vi "oa_TV Decimate N (NChan).vi"(5 "reset? (F)":bool, 8 "error in (no error)":errorcluster, 10 "pulse/revolution":i32[](array[numeric]), 11 "pulse position [s]":cluster{dbl[]}[](array[cluster]) {"?" format="%.2f"}) -> (0 "error out":errorcluster, 1 "revulotion index":i32[](array[numeric]), 2 "revulotion":i32[](array[numeric]), 3 "pulse positions":cluster{dbl[]}[](array[cluster]))   [LabVIEW 2017, in "SoundVib_Torsional.lvlib"]
uses:
  <vilib>/addons/Sound and Vibration/Order Analysis/Torsional Vibration/SoundVib_Torsional.lvlib
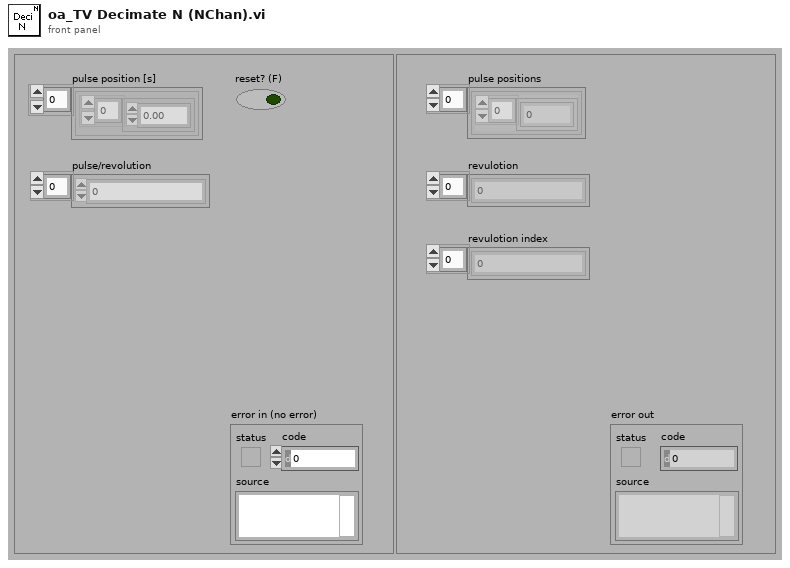
[diagram p1: front panel]
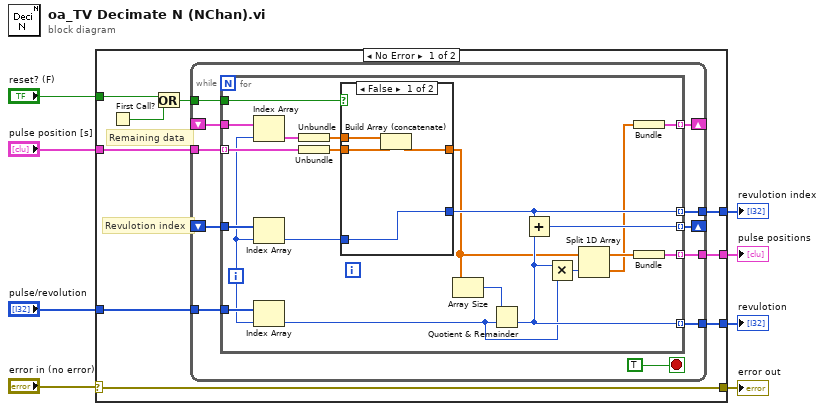
[diagram p0: block diagram]
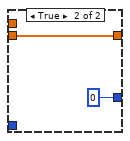
[diagram p2: hidden frame]
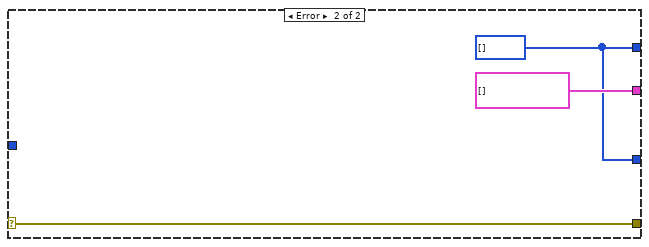
[diagram p3: hidden frame]
diagram:
  n1 = case shown="No Error" "error in (no error)" {
    selector: "error in (no error)" -> [w17 w58]
    tunnel: [w17 w58] -> w7
    tunnel: "pulse/revolution" -> [w16 _]
    tunnel: [w12 cluster{dbl[]}[] []] -> w5
    tunnel: [w15 w56] -> w4
    tunnel: "pulse position [s]" -> [w11 _]
    tunnel: [w10 w56] -> w2
    tunnel: "reset? (F)" -> [w9 _]
    frame No Error {
      # "Revulotion index"
      # "Remaining data"
      n2 = First Call?() -> (First Call?: T/F=w14:bool)
      n3 = Or(x=w9, y=w14) -> (x .or. y?=w13:bool)
      n4 = while {
        tunnel: w16 -> [w23]
        tunnel: [w24] -> w15
        tunnel: w13 -> [w28]
        shift-right: [w18] -> _
        shift-left: _ -> [w27]
        shift-right: [w26] -> _
        shift-left: _ -> [w25]
        tunnel: [w22] -> w12
        tunnel: [w21] -> w10
        tunnel: w11 -> [w19]
        stop <- TRUE stop-if-true
        n5 = for {
          tunnel: w28 -> [w48]
          tunnel: w19 -> [w43] mode=indexing
          tunnel: w27 -> [w38]
          tunnel: [w47] -> w26 mode=indexing
          tunnel: w25 -> [w37]
          tunnel: [w46] -> w24 mode=indexing
          tunnel: [w31] -> w18 mode=indexing
          tunnel: w23 -> [w36]
          tunnel: [w39] -> w22 mode=indexing
          tunnel: [w44] -> w21 mode=indexing
          i -> [w34]
          n6 = Index Array(array=w38, index=w34) -> (element=w30:cluster{dbl[]})
          n7 = Index Array(array=w37, index=w34) -> (element=w33:i32)
          n8 = Index Array(array=w36, index=w34) -> (element=w35:i32)
          n9 = Unbundle(w30) -> (w29:dbl[])
          n10 = Unbundle(w43) -> (w42:dbl[])
          n11 = case shown="False" w48 {
            tunnel: w29 -> [w51 _]
            tunnel: w33 -> [w53 _]
            tunnel: [w53 0] -> w46
            tunnel: w42 -> [w52 w54]
            tunnel: [w50 w54] -> w41
            frame False {
              n12 = Build Array (concatenate)(w51, w52) -> (w50:dbl[])
            }
            frame True {
            }
          }
          n13 = Array Size(array=w41) -> (size(s)=w49:i32)
          n14 = Quotient & Remainder(x=w49, y=w35) -> (floor(x/y)=w44:i32)  [unwired: 1 out]
          n15 = Add(x=w46, y=w44) -> (x+y=w47:i32)
          n16 = Multiply(x=w44, y=w35) -> (x*y=w45:i32)
          n17 = Split 1D Array(array=w41, index=w45) -> (first subarray=w40:dbl[], second subarray=w32:dbl[])
          n18 = Bundle(w32) -> (w31:cluster{dbl[]})  [unwired: 1 in]
          n19 = Bundle(w40) -> (w39:cluster{dbl[]})  [unwired: 1 in]
        }
      }
    }
    frame Error {
      w56 = i32[] []
    }
  }
  "error out" <- w7
  "pulse positions" <- w5
  "revulotion index" <- w4
  "revulotion" <- w2
